vi "Read LabVIEW version.vi"(8 "error in (no error)":errorcluster, 11 "LV DEV in":refnum<class "LV DEV.lvclass">) -> (0 "error out":errorcluster, 2 "LabVIEW version":string, 3 "LV DEV out":refnum<class "LV DEV.lvclass">)   [LabVIEW 2016, in "LV DEV.lvclass"]
uses:
  LV DEV.lvclass
  LV DEV.lvclass/LV DEV.ctl
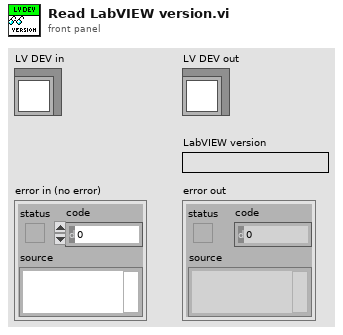
[diagram p1: front panel]
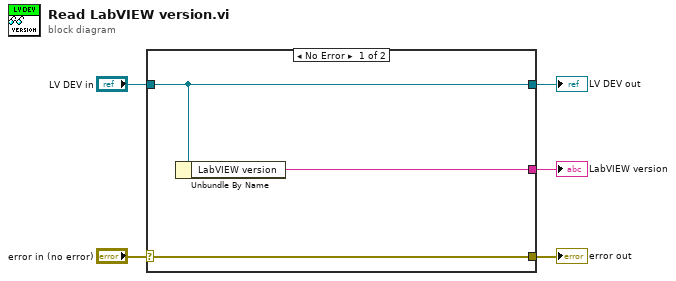
[diagram p0: block diagram]
diagram:
  n1 = case shown="No Error" "error in (no error)" {
    selector: "error in (no error)" -> [w8 w9]
    tunnel: [w8 w9] -> w4
    tunnel: [w7 w10] -> w2
    tunnel: "LV DEV in" -> [w7 w10]
    tunnel: [w6 _] -> w1
    frame No Error {
      n2 = Unbundle By Name(w7) -> ("LabVIEW version"=w6:string)
    }
    frame Error {
    }
  }
  "error out" <- w4
  "LV DEV out" <- w2
  "LabVIEW version" <- w1
